vi "Get KFMparam from PGserver.vi"(6 "conninfo":T4={"host"="localhost", "port"="5432", "client_encoding"="WIN1251", "dbname"="data", "user"="postgres", "password"=""}, 8 "error in (no error)":errorcluster, 9 "KFMParamColumns":string[](array[string])=["MVIName", "ip_adress", "port", "connection_timeout", "reconnection_timeout", "n_attempt_max", "reset_connect_timeout", "write_timeout", "read_timeout", "period", "enable", "write_enable", "fcode_full"], 10 "KFMParamTable":string="kfm_3", 11 "KFMParameters":string[](array[string])) -> (0 "error out":errorcluster, 1 "timeouts":T1[](array[typedef]), 2 "IP Address":T2(array[cluster]), 3 "MVIName":string[](array[string]), 4 "enable":bool[][](array[boolean]))   [LabVIEW 2019, in "ICPCON_Param.lvlib"]
uses:
  ICPCON_Param.lvlib
  Database/ctl/Coninfo.ctl
  Eth timeouts.ctl
  Database/PostgreSQL2LabVIEW/libpqlv/src/PQfinish.vi
  Database/PostgreSQL2LabVIEW/libpqlv/src/PQconnectdb.vi
  Database/PostgreSQL2LabVIEW/libpqlv/src/PQerrorMessage.vi
  Database/PostgreSQL2LabVIEW/libpqlv/src/PQstatus.vi
  <vilib>/dlg_ctls.llb/Space Constant.vi
  Database/PostgreSQL2LabVIEW/libpqUtility/libpqutility.lvlib
  Database/PostgreSQL2LabVIEW/libpqUtility64/libpqutility64.lvlib
  Database/PostgreSQL.lvlib
panel:
  out "progress 3":i32
  out "progress 2":i32
  out "PQStatus":T3(ring)
  # "fcode_full"
  # "fname"
  # "process_unit"
  # "port"
  # "connection_timeout"
  # "n_attempt_max"
  # "process_low_acd"
  # "instrument_range_max"
  # "d"
  # "input_register_min"
  # "input_register_max"
  # "input_pv_min"
  # "input_pv_max"
  # "ip_adress"
  # "fcodef"
  # "instrument_max_offset"
  # "reconnection_timeout"
  # "control_channel_num"
  # "process_range_max"
  # "process_high_acd"
  # "process_high_alr"
  # "process_low_alr"
  # "module_num"
  # "MVIName"
  # "ip_adress"
  # "fcode"
  # "Names"
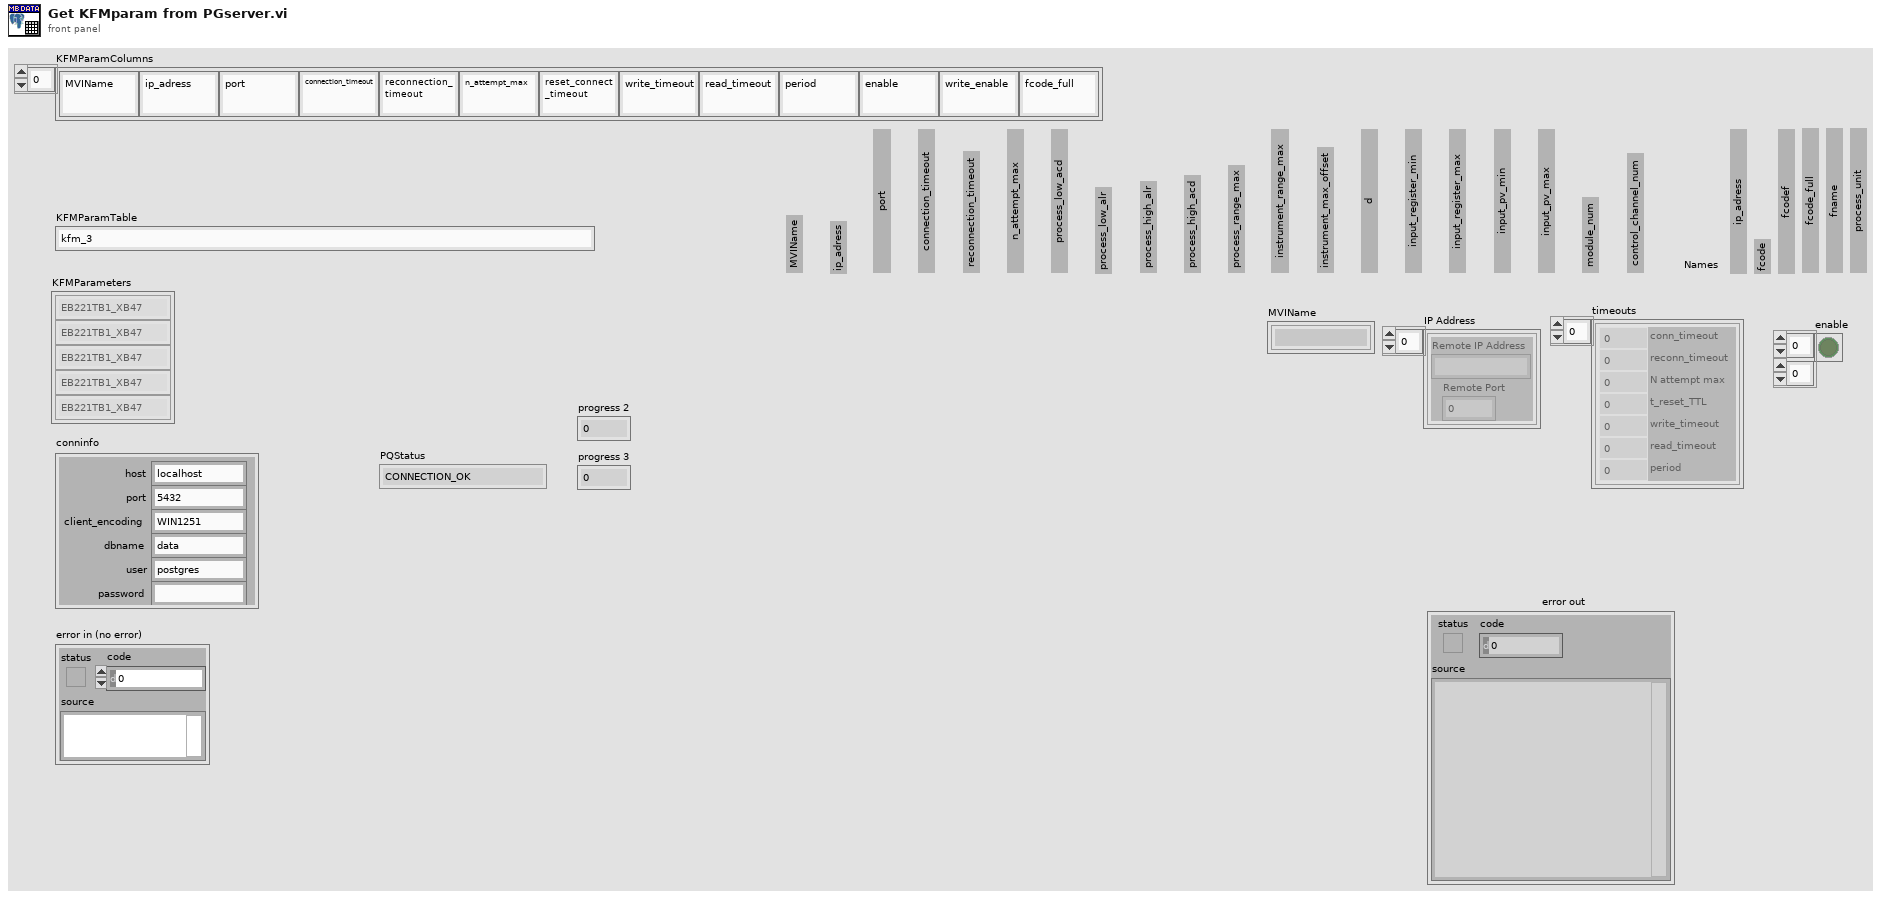
[diagram p1: front panel]
types:
  T1 = typedef "ICPCON_Param.lvlib/Eth timeouts.ctl" = cluster{"conn_timeout":i32, "reconn_timeout":i32, "N attempt max":i32, "t_reset_TTL":i32, "write_timeout":i32, "read_timeout":i32, "period":i32}
  T2 = cluster{"Remote IP Address":string, "Remote Port":u16}[]
  T3 = enum32{"CONNECTION_OK", "CONNECTION_BAD", "CONNECTION_STARTED", "CONNECTION_MADE", "CONNECTION_AWAITING_RESPONSE", "CONNECTION_AUTH_OK", "CONNECTION_SETENV", "CONNECTION_SSL_STARTUP", "CONNECTION_NEEDED"}
  T4 = typedef "PostgreSQL.lvlib/Coninfo.ctl" = cluster{"host":string, "port":string, "client_encoding":string, "dbname":string, "user":string, "password":string}
  T5 = cluster{"Remote IP Address":string, "Remote Port":u16}
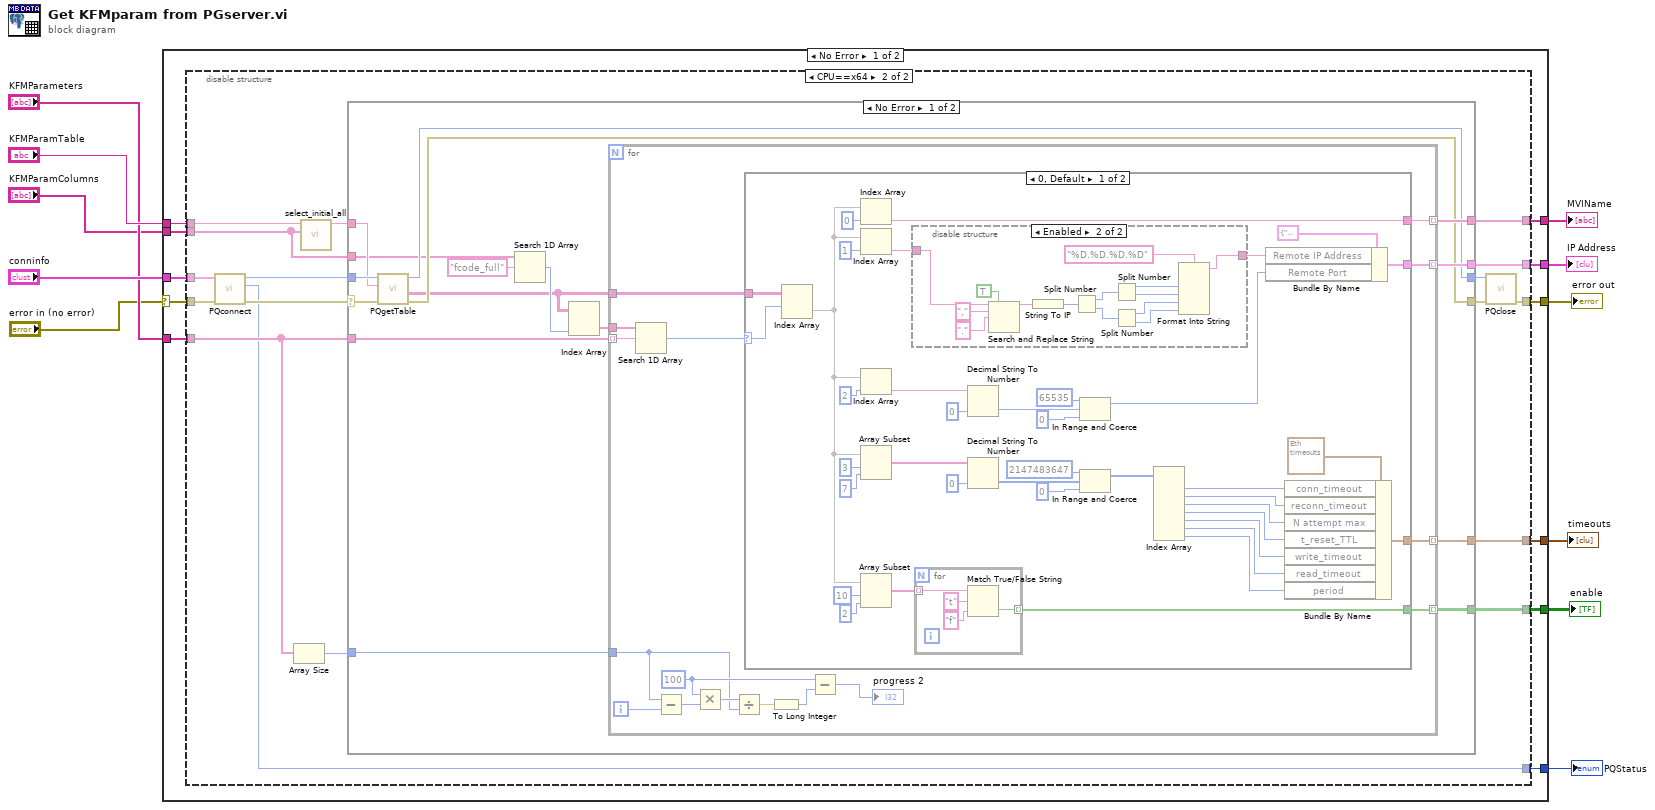
[diagram p0: block diagram]
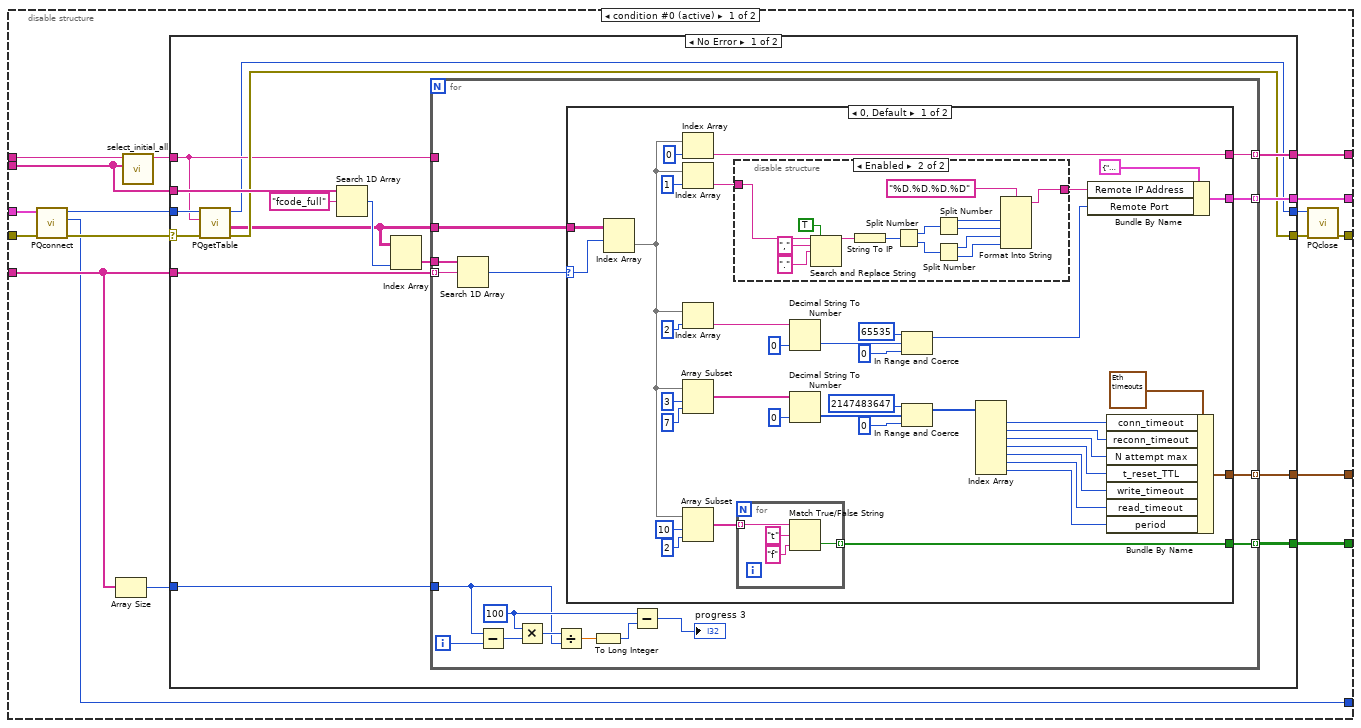
[diagram p2: hidden frame]
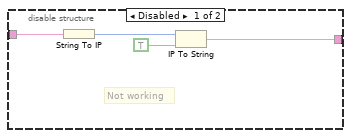
[diagram p3: hidden frame]
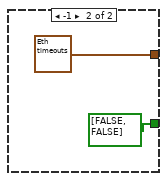
[diagram p4: hidden frame]
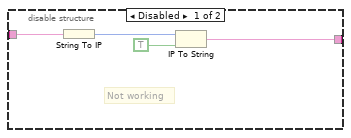
[diagram p6: hidden frame]
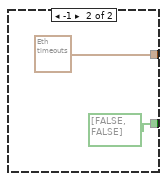
[diagram p7: hidden frame]
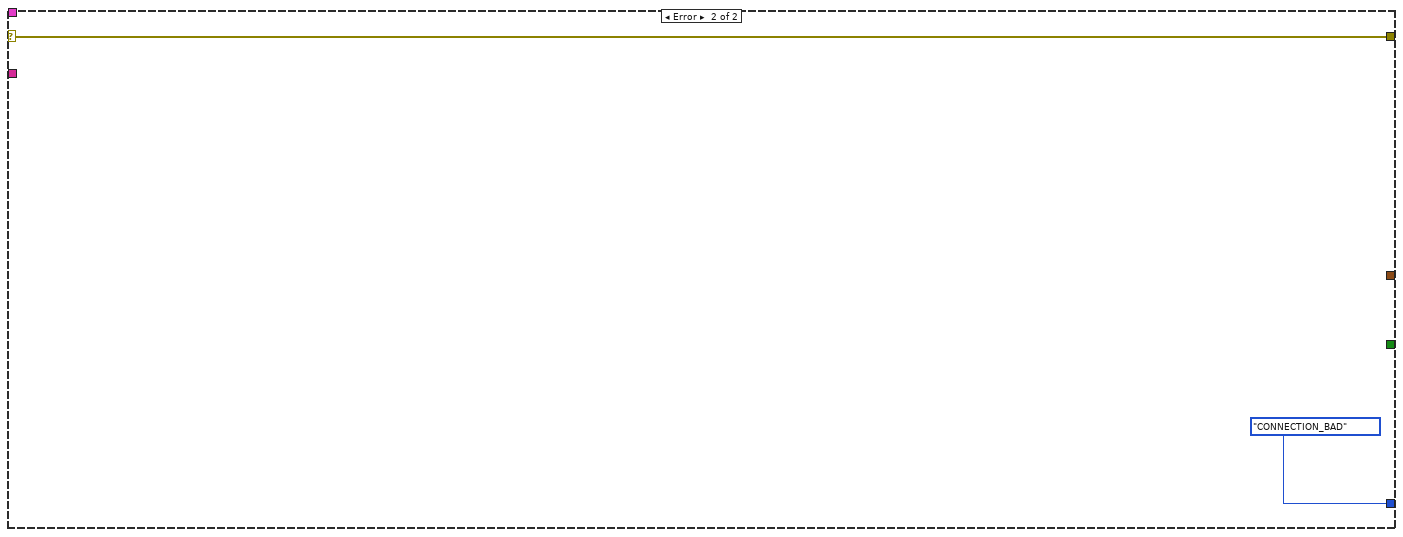
[diagram p9: hidden frame]
diagram:
  n1 = case shown="No Error" "error in (no error)" {
    selector: "error in (no error)" -> [w17 w250]
    tunnel: [w22 w250] -> w11
    tunnel: "KFMParamColumns" -> [w21 _]
    tunnel: "conninfo" -> [w20 _]
    tunnel: "KFMParamTable" -> [w19 _]
    tunnel: "KFMParameters" -> [w18 _]
    tunnel: [w16 T3."CONNECTION_BAD" ("PQStatus")] -> w6
    tunnel: [w15 _] -> w4
    tunnel: [w14 _] -> w3
    tunnel: [w13 _] -> w2
    tunnel: [w12 _] -> w1
    frame No Error {
      n2 = disable-structure shown="CPU==x64" {
        disable-tunnel: [w28 w139] -> w22
        disable-tunnel: w21 -> [w36 w136]
        disable-tunnel: w20 -> [w34 w144]
        disable-tunnel: w19 -> [w37 w138]
        disable-tunnel: w18 -> [w35 w152]
        disable-tunnel: w17 -> [w33 w146]
        disable-tunnel: [w30 w142] -> w16
        disable-tunnel: [w26 w149] -> w15
        disable-tunnel: [w25 w150] -> w14
        disable-tunnel: [w23 w151] -> w13
        disable-tunnel: [w24 w147] -> w12
        frame condition #0 (active) {
          n3 = call "PQconnect.vi"("error in (no error)"=w33, "conninfo"=w34) -> ("error out"=w31:errorcluster, "PQStatus"=w30:T3, "conn"=w32:u32)  [unwired: 7 in]
          n4 = Array Size(array=w35) -> (size(s)=w39:i32)
          n5 = call "select_initial_all.vi"("Column table"=w36, "table"=w37) -> ("parameters"=w38:string)  [unwired: 8 in, 1 out]
          n6 = case shown="No Error" w31 {
            selector: w31 -> [w40 w135]
            tunnel: w35 -> [w54 _]
            tunnel: w39 -> [w55 _]
            tunnel: w32 -> [w44 w134]
            tunnel: w38 -> [w43 _]
            tunnel: [w45 w135] -> w29
            tunnel: [w42 w134] -> w27
            tunnel: [w53 _] -> w26
            tunnel: [w52 _] -> w25
            tunnel: [w51 _] -> w23
            tunnel: [w50 _] -> w24
            tunnel: w36 -> [w46 _]
            frame No Error {
              n7 = call "PQgetTable.vi"("error in"=w40, "query"=w43, "conn"=w44) -> ("error out"=w45:errorcluster, "Data"=w41:string[][], "conn_out"=w42:u32)  [unwired: 4 in, 2 out]
              n8 = Search 1D Array(1D array=w46, element="fcode_full" ("table")) -> (index of element=w48:i32)  [unwired: 1 in]
              n9 = Index Array(array=w41, index (col)=w48) -> (element=w47:string[])  [unwired: 1 in]
              n10 = for {
                tunnel: w55 -> [w65]
                tunnel: w54 -> [w57] mode=indexing
                tunnel: w43 -> [_]
                tunnel: [w63] -> w53 mode=indexing
                tunnel: [w62] -> w52 mode=indexing
                tunnel: [w61] -> w51 mode=indexing
                tunnel: [w60] -> w50 mode=indexing
                tunnel: w41 -> [w59]
                tunnel: w47 -> [w58]
                i -> [w66]
                w70 = 100 ("y")
                n11 = Search 1D Array(1D array=w58, element=w57) -> (index of element=w56:i32)  [unwired: 1 in]
                n12 = Subtract(x=w65, y=w66) -> (x-y=w69:i32)
                n13 = Multiply(x=w70, y=w69) -> (x*y=w71:i32)
                n14 = Divide(x=w71, y=w65) -> (x/y=w68:dbl)
                n15 = case shown="0, Default" w56 {
                  selector: w56 -> [w76 _]
                  tunnel: [w108 _] -> w63
                  tunnel: [w90 bool[] [FALSE, FALSE]] -> w61
                  tunnel: [w89 _] -> w62
                  tunnel: [w79 T1 {"conn_timeout"=1000, "reconn_timeout"=3000, "N attempt max"=3, "t_reset_TTL"=120000, "write_timeout"=50, "read_timeout"=500, "period"=100} ("timeouts")] -> w60
                  tunnel: w59 -> [w78 _]
                  frame 0, Default {
                    n16 = Index Array(array=w78, index (row)=w76) -> (element=w92:string[])  [unwired: 1 in]
                    n17 = Index Array(array=w92, index=0) -> (element=w108:string)
                    n18 = Index Array(array=w92, index=1) -> (element=w107:string)
                    n19 = Index Array(array=w92, index=2) -> (element=w103:string)
                    n20 = Array Subset(array=w92, index=3, length=7 ("y")) -> (w95:string[])
                    n21 = Array Subset(array=w92, index=10, length=2) -> (w91:string[])
                    n22 = disable-structure shown="Enabled" {
                      disable-tunnel: w107 -> [w113 w115]
                      disable-tunnel: [w112 w114] -> w101
                      frame Disabled {
                        # "Not working"
                        n23 = String To IP(1:w113) -> (0:w111:u32)
                        n24 = IP To String(1:TRUE ("dot notation? (F)"), 2:w111) -> (0:w112:string)
                      }
                      frame Enabled {
                        n25 = Search and Replace String(replace all?=TRUE ("replace all? (F)"), input string=w115, search string=",", replace string="." ("replace string (\"\")")) -> (result string=w117:string)  [unwired: 4 in, 3 out]
                        n26 = String To IP(1:w117) -> (0:w127:u32)
                        n27 = Split Number(x=w127) -> (hi(x)=w126:u16, lo(x)=w125:u16)
                        n28 = Split Number(x=w126) -> (hi(x)=w123:u8, lo(x)=w122:u8)
                        n29 = Split Number(x=w125) -> (hi(x)=w121:u8, lo(x)=w120:u8)
                        n30 = Format Into String(format string="%D.%D.%D.%D", w123, w122, w121, w120) -> (resulting string=w114:string)  [unwired: 2 in, 1 out]
                      }
                    }
                    n31 = for {
                      tunnel: w91 -> [w130] mode=indexing
                      tunnel: [w128] -> w90 mode=indexing
                      n32 = Match True/False String(2:"f" ("false string"), 3:"t" ("true string"), 4:w130) -> (0:w128:bool)  [unwired: 1 out]
                    }
                    n33 = Decimal String To Number(string=w103, default (0L)=0 ("default (0 I32)")) -> (number=w100:i32)  [unwired: 1 in, 1 out]
                    n34 = Decimal String To Number(string=w95, default (0L)=0 ("default (0 I32)")) -> (number=w72:i32[])  [unwired: 1 in, 1 out]
                    n35 = In Range and Coerce(upper limit=65535, x=w100, lower limit=0) -> (coerced(x)=w97:i32)  [unwired: 1 out]
                    n36 = In Range and Coerce(upper limit=2147483647, x=w72, lower limit=0) -> (coerced(x)=w80:i32[])  [unwired: 1 out]
                    n37 = Index Array(array=w80) -> (element #1=w87:i32, element #2=w86:i32, element #3=w85:i32, element #4=w84:i32, element #5=w83:i32, element #6=w82:i32, element #7=w81:i32)  [unwired: 7 in]
                    n38 = Bundle By Name(cluster=T5 {"Remote IP Address"="", "Remote Port"=502} ("IP address"), "Remote IP Address"=w101, "Remote Port"=w97) -> (w89:T5)
                    n39 = Bundle By Name(cluster=T1 {"conn_timeout"=1000, "reconn_timeout"=3000, "N attempt max"=3, "t_reset_TTL"=120000, "write_timeout"=50, "read_timeout"=500, "period"=100} ("timeouts"), "conn_timeout"=w87, "reconn_timeout"=w86, "N attempt max"=w85, "t_reset_TTL"=w84, "write_timeout"=w83, "read_timeout"=w82, "period"=w81) -> (w79:T1)
                  }
                  frame -1 {
                  }
                }
                n40 = To Long Integer(number=w68) -> (32bit integer=w67:i32)
                n41 = Subtract(x=w70, y=w67) -> (x-y=→"progress 3":i32)
              }
            }
            frame Error {
            }
          }
          n42 = call "PQclose.vi"("error in (no error)"=w29, "conn"=w27) -> ("error out"=w28:errorcluster)  [unwired: 9 in]
        }
        frame condition #1 {
          n43 = call "PQconnect.vi"("error in (no error)"=w146, "conninfo"=w144) -> ("error out"=w145:errorcluster, "PQStatus"=w142:T3, "conn"=w143:u64)  [unwired: 7 in]
          n44 = Array Size(array=w152) -> (size(s)=w148:i32)
          n45 = call "select_initial_all.vi"("Column table"=w136, "table"=w138) -> ("parameters"=w137:string)  [unwired: 8 in, 1 out]
          n46 = case shown="No Error" w145 {
            selector: w145 -> [w162 w248]
            tunnel: w152 -> [w167 _]
            tunnel: w148 -> [w168 _]
            tunnel: w143 -> [w161 w247]
            tunnel: w137 -> [w159 _]
            tunnel: [w160 w248] -> w140
            tunnel: [w155 w247] -> w141
            tunnel: [w166 _] -> w149
            tunnel: [w165 _] -> w150
            tunnel: [w164 _] -> w151
            tunnel: [w163 _] -> w147
            tunnel: w136 -> [w153 _]
            frame No Error {
              n47 = call "PQgetTable.vi"("error in"=w162, "query"=w159, "conn"=w161) -> ("error out"=w160:errorcluster, "Data"=w156:string[][], "conn_out"=w155:u64)  [unwired: 4 in, 2 out]
              n48 = Search 1D Array(1D array=w153, element="fcode_full" ("table")) -> (index of element=w157:i32)  [unwired: 1 in]
              n49 = Index Array(array=w156, index (col)=w157) -> (element=w154:string[])  [unwired: 1 in]
              n50 = for {
                tunnel: w168 -> [w178]
                tunnel: w167 -> [w170] mode=indexing
                tunnel: [w176] -> w166 mode=indexing
                tunnel: [w175] -> w165 mode=indexing
                tunnel: [w174] -> w164 mode=indexing
                tunnel: [w173] -> w163 mode=indexing
                tunnel: w156 -> [w172]
                tunnel: w154 -> [w171]
                i -> [w179]
                w183 = 100 ("y")
                n51 = Search 1D Array(1D array=w171, element=w170) -> (index of element=w169:i32)  [unwired: 1 in]
                n52 = Subtract(x=w178, y=w179) -> (x-y=w182:i32)
                n53 = Multiply(x=w183, y=w182) -> (x*y=w184:i32)
                n54 = Divide(x=w184, y=w178) -> (x/y=w181:dbl)
                n55 = case shown="0, Default" w169 {
                  selector: w169 -> [w189 _]
                  tunnel: [w221 _] -> w176
                  tunnel: [w203 bool[] [FALSE, FALSE]] -> w174
                  tunnel: [w202 _] -> w175
                  tunnel: [w192 T1 {"conn_timeout"=1000, "reconn_timeout"=3000, "N attempt max"=3, "t_reset_TTL"=120000, "write_timeout"=50, "read_timeout"=500, "period"=100} ("timeouts")] -> w173
                  tunnel: w172 -> [w191 _]
                  frame 0, Default {
                    n56 = Index Array(array=w191, index (row)=w189) -> (element=w205:string[])  [unwired: 1 in]
                    n57 = Index Array(array=w205, index=0) -> (element=w221:string)
                    n58 = Index Array(array=w205, index=1) -> (element=w220:string)
                    n59 = Index Array(array=w205, index=2) -> (element=w216:string)
                    n60 = Array Subset(array=w205, index=3, length=7 ("y")) -> (w208:string[])
                    n61 = Array Subset(array=w205, index=10, length=2) -> (w204:string[])
                    n62 = disable-structure shown="Enabled" {
                      disable-tunnel: w220 -> [w226 w228]
                      disable-tunnel: [w225 w227] -> w214
                      frame Disabled {
                        # "Not working"
                        n63 = String To IP(1:w226) -> (0:w224:u32)
                        n64 = IP To String(1:TRUE ("dot notation? (F)"), 2:w224) -> (0:w225:string)
                      }
                      frame Enabled {
                        n65 = Search and Replace String(replace all?=TRUE ("replace all? (F)"), input string=w228, search string=",", replace string="." ("replace string (\"\")")) -> (result string=w230:string)  [unwired: 4 in, 3 out]
                        n66 = String To IP(1:w230) -> (0:w240:u32)
                        n67 = Split Number(x=w240) -> (hi(x)=w239:u16, lo(x)=w238:u16)
                        n68 = Split Number(x=w239) -> (hi(x)=w236:u8, lo(x)=w235:u8)
                        n69 = Split Number(x=w238) -> (hi(x)=w234:u8, lo(x)=w233:u8)
                        n70 = Format Into String(format string="%D.%D.%D.%D", w236, w235, w234, w233) -> (resulting string=w227:string)  [unwired: 2 in, 1 out]
                      }
                    }
                    n71 = for {
                      tunnel: w204 -> [w243] mode=indexing
                      tunnel: [w241] -> w203 mode=indexing
                      n72 = Match True/False String(2:"f" ("false string"), 3:"t" ("true string"), 4:w243) -> (0:w241:bool)  [unwired: 1 out]
                    }
                    n73 = Decimal String To Number(string=w216, default (0L)=0 ("default (0 I32)")) -> (number=w213:i32)  [unwired: 1 in, 1 out]
                    n74 = Decimal String To Number(string=w208, default (0L)=0 ("default (0 I32)")) -> (number=w185:i32[])  [unwired: 1 in, 1 out]
                    n75 = In Range and Coerce(upper limit=65535, x=w213, lower limit=0) -> (coerced(x)=w210:i32)  [unwired: 1 out]
                    n76 = In Range and Coerce(upper limit=2147483647, x=w185, lower limit=0) -> (coerced(x)=w193:i32[])  [unwired: 1 out]
                    n77 = Index Array(array=w193) -> (element #1=w200:i32, element #2=w199:i32, element #3=w198:i32, element #4=w197:i32, element #5=w196:i32, element #6=w195:i32, element #7=w194:i32)  [unwired: 7 in]
                    n78 = Bundle By Name(cluster=T5 {"Remote IP Address"="", "Remote Port"=502} ("IP address"), "Remote IP Address"=w214, "Remote Port"=w210) -> (w202:T5)
                    n79 = Bundle By Name(cluster=T1 {"conn_timeout"=1000, "reconn_timeout"=3000, "N attempt max"=3, "t_reset_TTL"=120000, "write_timeout"=50, "read_timeout"=500, "period"=100} ("timeouts"), "conn_timeout"=w200, "reconn_timeout"=w199, "N attempt max"=w198, "t_reset_TTL"=w197, "write_timeout"=w196, "read_timeout"=w195, "period"=w194) -> (w192:T1)
                  }
                  frame -1 {
                  }
                }
                n80 = To Long Integer(number=w181) -> (32bit integer=w180:i32)
                n81 = Subtract(x=w183, y=w180) -> (x-y=→"progress 2":i32)
              }
            }
            frame Error {
            }
          }
          n82 = call "PQclose.vi"("error in (no error)"=w140, "conn"=w141) -> ("error out"=w139:errorcluster)  [unwired: 9 in]
        }
      }
    }
    frame Error {
    }
  }
  "error out" <- w11
  "PQStatus" <- w6
  "MVIName" <- w4
  "enable" <- w2
  "IP Address" <- w3
  "timeouts" <- w1
